vi "Log info.vi"(6 "Ref ?":bool, 7 "Rows":i32=50, 8 "error in (no error)":errorcluster caption="错误输入（无错误）", 9 "information":T1, 10 "MCListbox引用句柄":refnum<vi>, 11 "Base":path) -> (0 "error out":errorcluster caption="错误输出", 3 "MCListbox":refnum<vi>)   [LabVIEW 2014]
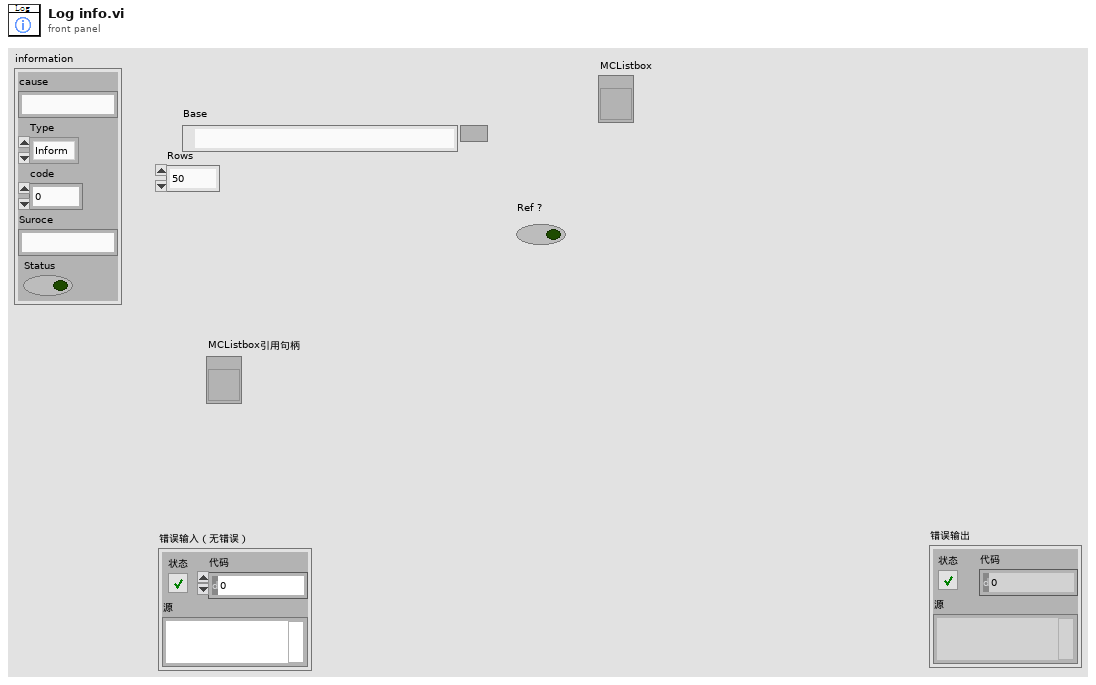
[diagram p1: front panel]
types:
  T1 = cluster{"cause":string, "Type":enum16{"Inform", "Warning", "Alarm"}, "code":i32, "Suroce":string, "Status":bool}
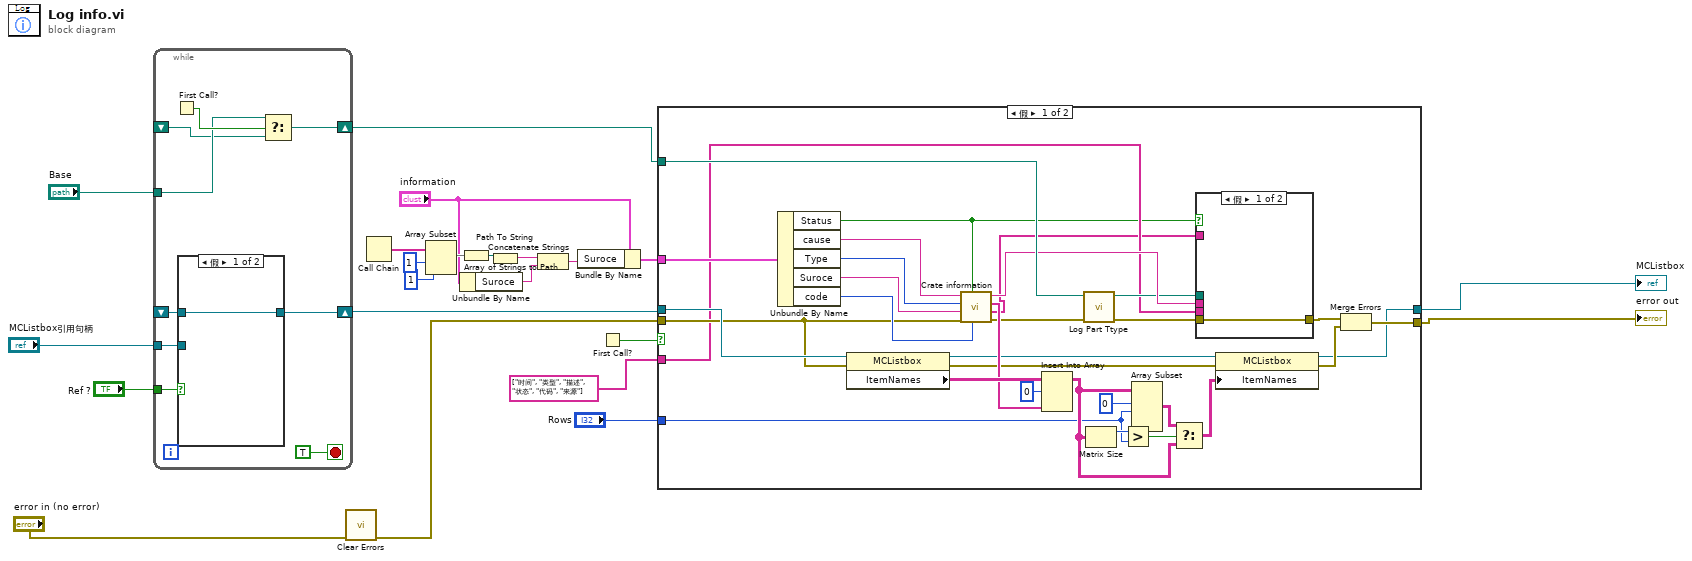
[diagram p0: block diagram]
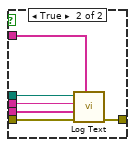
[diagram p3: hidden frame]
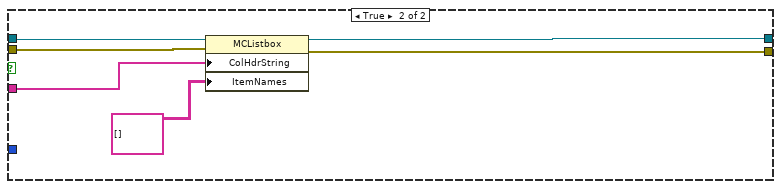
[diagram p4: hidden frame]
diagram:
  n1 = while {
    tunnel: "Ref ?" -> [w30]
    shift-right: [w29] -> w12
    shift-left: _ -> [w28]
    tunnel: "MCListbox引用句柄" -> [w27]
    shift-right: [w26] -> w6
    shift-left: _ -> [w23]
    tunnel: "Base" -> [w24]
    stop <- TRUE stop-if-true
    n2 = First Call?() -> (First Call?: T/F=w25:bool)
    n3 = case shown="假" w30 {
      tunnel: [w32 w33] -> w29
      tunnel: w28 -> [w32 _]
      tunnel: w27 -> [_ w33]
      frame False {
      }
      frame True {
      }
    }
    n4 = Select(t=w24, s=w25, f=w23) -> (s? t:f=w26:path)
  }
  n5 = call <vilib>:"Clear Errors.vi"("error in (no error)"="error in (no error)") -> ("error out"=w2:errorcluster)  [unwired: 5 in, 1 out]
  n6 = Call Chain() -> (call chain=w18:string[])
  n7 = Array Subset(array=w18, index=1 ("索引"), length=1 ("长度")) -> (w16:string[])
  n8 = Unbundle By Name("information") -> ("Suroce"=w7:string)
  n9 = Array of Strings to Path(0:w16) -> (2:w15:path)  [unwired: 1 in]
  n10 = Path To String(path=w15) -> (string=w9:string)
  n11 = Concatenate Strings(w9, w7) -> (w8:string)
  n12 = Bundle By Name(cluster="information", "Suroce"=w8) -> (w19:T1)
  n13 = First Call?() -> (First Call?: T/F=w1:bool)
  n14 = case shown="假" w1 {
    tunnel: w12 -> [w59 w77]
    tunnel: w2 -> [w58 w76]
    tunnel: string[] ["时间", "类型", "描述", "状态", "代码", "来源"] -> [w43 w75]
    tunnel: [w44 w73] -> w21
    tunnel: w19 -> [w60 _]
    tunnel: w6 -> [w50 _]
    tunnel: [w45 w72] -> w20
    tunnel: "Rows" -> [w36 _]
    frame False {
      n15 = Unbundle By Name(w60) -> ("Status"=w34:bool, "cause"=w61:string, "Type"=w62:enum16{"Inform", "Warning", "Alarm"}, "Suroce"=w63:string, "code"=w64:i32)
      n16 = property class="MCListbox"(reference=w59, error in=w58) -> (reference out=w54:refnum<vi>, error out=w53:errorcluster, "ItemNames"=w57:string[][])
      n17 = call "Crate information.vi"("code"=w64, "Status"=w34, "error in (no error)"=w58, "Suroce"=w63, "Type"=w62, "cause"=w61) -> ("error out"=w52:errorcluster, "appended array"=w35:string[], "Log Array"=w56:string[], "Log imform"=w49:string)  [unwired: 2 in]
      n18 = Insert Into Array(array=w57, index (row)=0 ("索引 (行)"), new element=w56) -> (w39:string[][])  [unwired: 1 in]
      n19 = call "Log Part Ttype.vi"("error in (no error)"=w52, "Base"=w50) -> ("error out"=w51:errorcluster, "添加的路径"=w48:path)  [unwired: 8 in]
      n20 = Matrix Size(0:w39) -> (1:w42:i32)  [unwired: 1 out]
      n21 = Greater?(x=w42, y=w36) -> (0:w41:bool)
      n22 = Array Subset(array=w39, index (row)=0 ("索引"), length (row)=w36) -> (w37:string[][])  [unwired: 2 in]
      n23 = Select(t=w37, s=w41, f=w39) -> (s? t:f=w40:string[][])
      n24 = case shown="假" w34 {
        tunnel: w51 -> [w65 w71]
        tunnel: w49 -> [_ w70]
        tunnel: w48 -> [_ w69]
        tunnel: [w65 w68] -> w47
        tunnel: w43 -> [_ w67]
        tunnel: w35 -> [_ w66]
        frame False {
        }
        frame True {
          n25 = call "Log Text.vi"("Log Array"=w66, "error in (no error)"=w71, "Hearder"=w67, "log text"=w70, "Path"=w69) -> ("error out"=w68:errorcluster)  [unwired: 5 in, 1 out]
        }
      }
      n26 = property class="MCListbox"(reference=w54, error in=w53, "ItemNames"=w40) -> (reference out=w44:refnum<vi>, error out=w46:errorcluster)
      n27 = Merge Errors(w47, w46) -> (w45:errorcluster)
    }
    frame True {
      n28 = property class="MCListbox"(reference=w77, error in=w76, "ColHdrString"=w75, "ItemNames"=string[][] [] ("项名")) -> (reference out=w73:refnum<vi>, error out=w72:errorcluster)
    }
  }
  "error out" <- w20
  "MCListbox" <- w21
